vi "ADS1015 Raw2Formatted Converter.vi"(10 "Gain (mV/bit)":dbl=0.003, 11 "Bytes Read":u8[](array[numeric]) format="%08b") -> (3 "Numeric Indicator":dbl)   [LabVIEW 2014]
panel:
  out "x << y":u16 format="%016b"
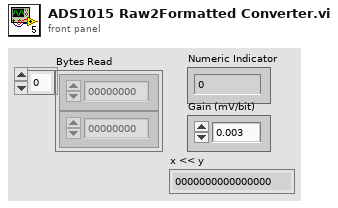
[diagram p1: front panel]
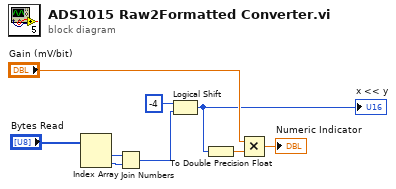
[diagram p0: block diagram]
diagram:
  n1 = Index Array(array="Bytes Read") -> (element #1=w5:u8, element #2=w4:u8)  [unwired: 2 in]
  n2 = Join Numbers(hi=w5, lo=w4) -> ((hi.lo)=w2:u16)
  n3 = Logical Shift(y=i16 -4 ("x"), x=w2) -> (x << y=w3:u16)
  "x << y" <- w3
  n4 = To Double Precision Float(number=w3) -> (double precision float=w9:dbl)
  n5 = Multiply(x="Gain (mV/bit)", y=w9) -> (x*y=→"Numeric Indicator":dbl)
